vi "SynapseAPI-Set Tank.vi"(0 "URL":string="http://localhost:24414", 7 "tank":string, 11 "error in (no error)":errorcluster) -> (15 "error out":errorcluster)   [LabVIEW 2020]
uses:
  <vilib>/httpClient/PUTBuffer.vi
  <vilib>/httpClient/LabVIEWHTTPClient.lvlib
panel:
  out "headers":string
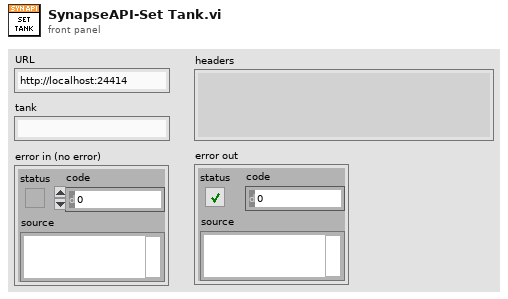
[diagram p1: front panel]
types:
  T1 = typedef "LabVIEWHTTPClient.lvlib/ClientHandle.ctl" = refnum<k1>
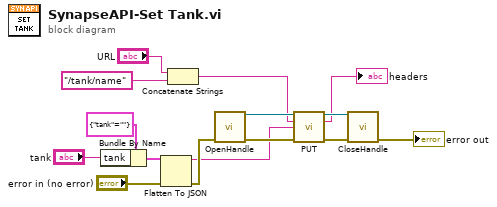
[diagram p0: block diagram]
diagram:
  n1 = Bundle By Name(cluster=cluster{"tank":string} {"tank"=""} ("Cluster"), "tank"="tank") -> (w14:cluster{"tank":string})
  n2 = Flatten To JSON(anything=w14, error in (no error)="error in (no error)") -> (JSON string=w5:string, 11:w6:errorcluster)  [unwired: 1 in]
  n3 = Concatenate Strings("URL", "/tank/name") -> (w7:string)
  n4 = call <vilib>:"OpenHandle.vi"("error in (no error)"=w6) -> ("client handle out"=w10:T1, "error out"=w9:errorcluster)  [unwired: 13 in]
  n5 = call-poly <vilib>:"PUT.vi"("client handle"=w10, "url"=w7, "buffer"=w5, "error in (no error)"=w9) -> ("client handle out"=w12:T1, "headers"=→"headers":string, "error out"=w13:errorcluster)  [unwired: 8 in, 1 out]
  n6 = call <vilib>:"CloseHandle.vi"("client handle"=w12, "error in (no error)"=w13) -> ("error out"=→"error out":errorcluster)  [unwired: 13 in]
